vi "RRI LoadGo - Electromagnet.vi"(5 "Control Coils":T1(ring), 6 "Hardware Parameters":T2={"Scan Calibration [G/V]"=0.0, "Modulation Calibration [G/V]"=0.0, "Modulation Phase [deg]"=0.0, "Modulation Frequency [Hz]"=0.0, "Attenuation [dB]"=0, "Input Channel Count"=0, "Time constant"=7, "Sensitivity"=17, "Frequency Output Voltage [V]"=0.0, "Phase Output Voltage [V]"=0.0, "Lock-in Offset Compensation"=FALSE, "RF [GHz]"=0.0, "Q Start"=0.0, "Q End"=0.0, "Balance"=0.0, "Phase Error"=0.0, "AFC Error"=0.0, "AFC"=FALSE, "Magnet Rotation"=FALSE, "Balance Scaling Factor"=1.0, "Phase Error Scaling Factor"=1.0, "AFC Error Scaling Factor"=1.0, "Frequency Counter ID"="", "Sweep Waveform"=enum."Sawtooth", "Q-Factor Scale"=0.0, " Q-Data Scale"=0.0, " Q-Data Offset"=0.0, "Magnet Rotation Slope"=0.0, "Magnet Rotation Offset"=0.0, "Phase Sweep Resolution"=0.0, "Hardware Version Number"="", "Spectrometer ID Number"=0, "Spectrometer Name"="", "Lock in Saturation"=0.0, "Balance Threshold"=0.0, "Phase Error Threshold"=0.0, "AFC Error Threshold"=0.0, "Linear Actuator Length"=0.0, "Lock-in OK?"=FALSE, "Ignore Lock-in Comm. Failure"=FALSE, "Gradient Addresses"=[], "Gradient Calibrations [G/A*mm]"=[], "Gradient Power Supplies"=[], "Lock-in Address"="", "Magnet Type"=enum."RRI", "Camera Names"=[], "Sweep Limit [Gauss]"=0.0, "Modulation Limit [Gauss]"=0.0, "Balance Threshold Exceeded?"=FALSE, "Phase Threshold Exceeded?"=FALSE, "AFC Threshold Exceeded?"=FALSE, "Consecutive Re-tune attempts"=0, "Reverse Sweep Slope [sec]"=0.0, "Reverse Sweep Offset [G]"=0.0, "AFC Field Correction [V/MHz]"=0.0, "Active Gradients (X Y Z)"=[], "SpO2 Calibration [SpO2/V]"=1.0, "Heart Rate Calibration [BPM/V]"=1.0, "Thermocouple Channel"=""} {"Sensitivity" items=["", "2 nV", "5 nV", "10 nV", "20 nV", "50 nV", "100 nV", "200 nV", "500 nV", "1 uV", "2 uV", "5 uV", "10 uV", "20 uV", "50 uV", "100 uV", "200 uV", "500 uV", "1 mV", "2 mV", "5 mV", "10 mV", "20 mV", "50 mV", "100 mV", "200 mV", "500 mV", "1 V"]; "Time constant" items=["10 us", "20 us", "40 us", "80 us", "160 us", "320 us", "640 us", "5 ms", "10 ms", "20 ms", "50 ms", "100 ms", "200 ms", "500 ms", "1 s", "2 s", "5 s", "10 s", "20 s", "50 s", "100 s", "200 s", "500 s", "1 ks", "2 ks", "5 ks", "10 ks", "20 ks", "50 ks", "100 ks"]}, 7 "Acquisition Parameters":T3={"Magnet Angle [deg]"=0.0, "Magnet Angles [deg]"=[], "DeltaVpp [v]"=0.0, "SEM [v]"=0.0, "DeltaVpp Thresh [v]"=0.0, "SEM Thresh [v]"=0.0, "Adaptive Processing"=FALSE, "Acquire Q"=FALSE, "Acquire Photos"=FALSE, "Adaptive Tuning"=FALSE, "Automated Matching"=FALSE, "X-Gradient [G/mm]"=0.0, "Y-Gradient [G/mm]"=0.0, "Z-Gradient [G/mm]"=0.0, "Central Field [G]"=0.0, "Scan Width [G]"=0.0, "Mod. Amp. [G]"=0.0, "Scan Time [s]"=0.0, "Pre-Scan Delay [ms]"=0, "Measurement Timeout [s]"=0.0, "Electromagnet Main Field [G]"=0.0, "Locked Central Field [G]"=0.0, "Scans Excluded"=0, "Scans Completed"=0, "No. Scans/Set"=0, "No. Scans for SNR"=0, "Field Locked Frequency [GHz]"=0.0, "Auto Set-based Field Center"=FALSE, "Prompt for oxy acquisition updates"=FALSE, "Oxy QA Scan?"=FALSE, "Exclude Bad Data"=FALSE, "Optimizing RF Power"=FALSE, "Gradients on/off"=FALSE, "Running Script"=TRUE, "Opto-Coupler Current [A]"=0.0, "Continuous Sweeping"=FALSE, "Sweep Rise Time [sec]"=0, "Reverse Sweep Central Field [G]"=0.0, "Forward Sweep Central Field [G]"=0.0, "Sweep Calibrated"=FALSE, "Modulation Calibrated"=FALSE, "First CheckCal Scan?"=FALSE, "AFC Field Correction"=FALSE, "OxyQAInit Scan Width [G]"=0.0, "OxyQAInit Mod. Amp. [G]"=0.0, "Scans Completed/Session"=0, "Acquire SpO2"=FALSE, "Acquire Temperature"=FALSE, "Over Mod"=FALSE} {"OxyQAInit Mod. Amp. [G]" min=0.0; "OxyQAInit Scan Width [G]" min=0.0; "Mod. Amp. [G]" min=0.0; "Scan Width [G]" min=0.0; "Measurement Timeout [s]" min=0.0; "Scan Time [s]" min=0.0; "Z-Gradient [G/mm]" min=0.0; "Y-Gradient [G/mm]" min=0.0; "X-Gradient [G/mm]" min=0.0; "SEM Thresh [v]" min=0.0; "DeltaVpp Thresh [v]" min=0.0; "SEM [v]" min=0.0}) -> (0 "error out":errorcluster)   [LabVIEW 2016]
uses:
  Types/Acquisition Parameters.ctl
  Types/Hardware Parameters.ctl
  <vilib>/Instr/_visa.llb/VISA Configure Serial Port (Instr).vi
panel:
  # "Bridge I/O"
  # "Magnet Rotation"
  # "Field Calibration"
  # "Lock In Amplifier"
  # "Spectrometer Information"
  # "DAQ Settings"
  # "Gradient Coils and Field"
  # "X"
  # "Y"
  # "Z"
  # "Q-Measurements"
  # "Gradients"
  # "Field"
  # "Scans and Sets"
  # "Timing"
  # "Adaptive Dosimetric \nData Processing"
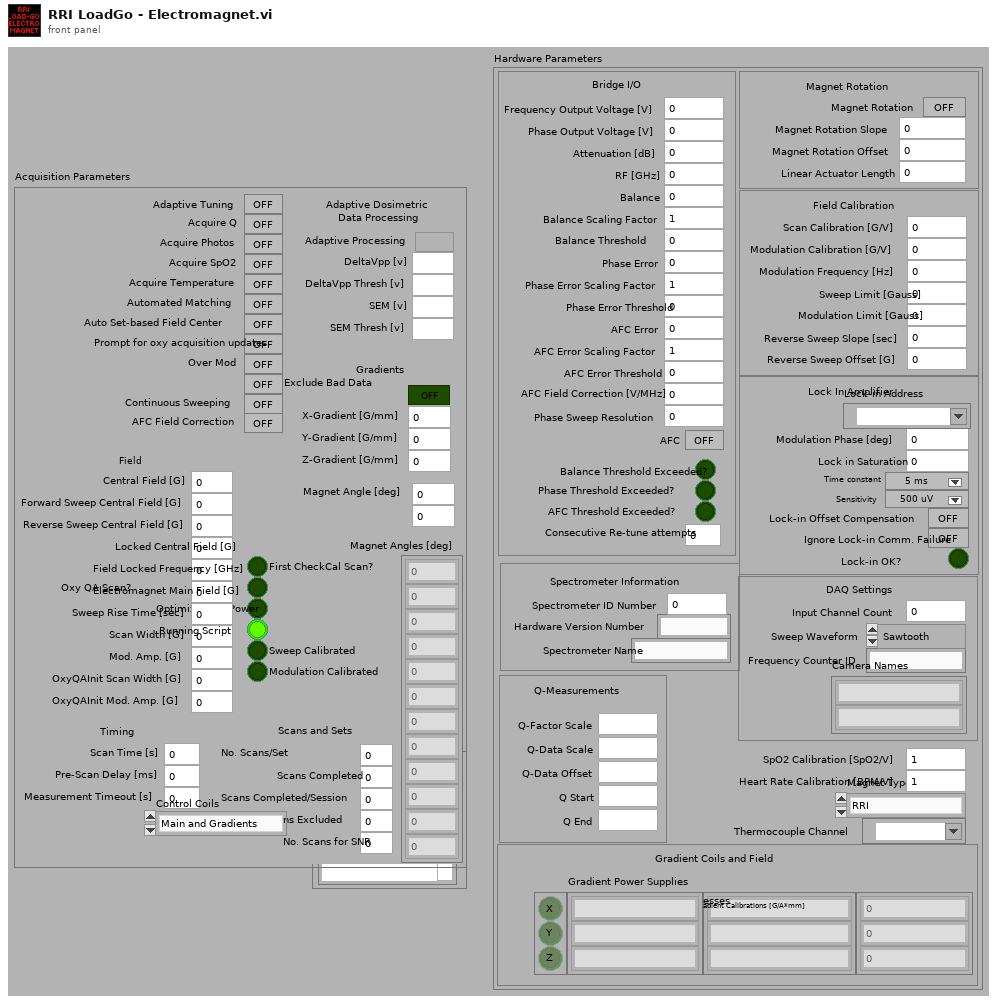
[diagram p1: front panel]
types:
  T1 = enum16{"Main and Gradients", "Main Field", "Gradients"}
  T2 = typedef "Hardware Parameters.ctl" = cluster{"Scan Calibration [G/V]":dbl, "Modulation Calibration [G/V]":dbl, "Modulation Phase [deg]":dbl, "Modulation Frequency [Hz]":dbl, "Attenuation [dB]":u16, "Input Channel Count":i32, "Time constant":u16, "Sensitivity":u16, "Frequency Output Voltage [V]":dbl, "Phase Output Voltage [V]":dbl, "Lock-in Offset Compensation":bool, "RF [GHz]":dbl, "Q Start":dbl, "Q End":dbl, "Balance":dbl, "Phase Error":dbl, "AFC Error":dbl, "AFC":bool, "Magnet Rotation":bool, "Balance Scaling Factor":dbl, "Phase Error Scaling Factor":dbl, "AFC Error Scaling Factor":dbl, "Frequency Counter ID":string, "Sweep Waveform":enum16{"Sine Wave", "Square Wave", "Sawtooth", "Triangle Wave"}, "Q-Factor Scale":dbl, " Q-Data Scale":dbl, " Q-Data Offset":dbl, "Magnet Rotation Slope":dbl, "Magnet Rotation Offset":dbl, "Phase Sweep Resolution":dbl, "Hardware Version Number":string, "Spectrometer ID Number":i32, "Spectrometer Name":string, "Lock in Saturation":dbl, "Balance Threshold":dbl, "Phase Error Threshold":dbl, "AFC Error Threshold":dbl, "Linear Actuator Length":dbl, "Lock-in OK?":bool, "Ignore Lock-in Comm. Failure":bool, "Gradient Addresses":string[], "Gradient Calibrations [G/A*mm]":dbl[], "Gradient Power Supplies":string[], "Lock-in Address":refnum<visa-resource-name>, "Magnet Type":enum16{"RRI", "BARDA", "Whole Body Permanent", "RRI Electromagnet"}, "Camera Names":string[], "Sweep Limit [Gauss]":dbl, "Modulation Limit [Gauss]":dbl, "Balance Threshold Exceeded?":bool, "Phase Threshold Exceeded?":bool, "AFC Threshold Exceeded?":bool, "Consecutive Re-tune attempts":i32, "Reverse Sweep Slope [sec]":dbl, "Reverse Sweep Offset [G]":dbl, "AFC Field Correction [V/MHz]":dbl, "Active Gradients (X Y Z)":bool[], "SpO2 Calibration [SpO2/V]":dbl, "Heart Rate Calibration [BPM/V]":dbl, "Thermocouple Channel":tag}
  T3 = typedef "Acquisition Parameters.ctl" = cluster{"Magnet Angle [deg]":dbl, "Magnet Angles [deg]":dbl[], "DeltaVpp [v]":dbl, "SEM [v]":dbl, "DeltaVpp Thresh [v]":dbl, "SEM Thresh [v]":dbl, "Adaptive Processing":bool, "Acquire Q":bool, "Acquire Photos":bool, "Adaptive Tuning":bool, "Automated Matching":bool, "X-Gradient [G/mm]":dbl, "Y-Gradient [G/mm]":dbl, "Z-Gradient [G/mm]":dbl, "Central Field [G]":dbl, "Scan Width [G]":dbl, "Mod. Amp. [G]":dbl, "Scan Time [s]":dbl, "Pre-Scan Delay [ms]":u32, "Measurement Timeout [s]":dbl, "Electromagnet Main Field [G]":dbl, "Locked Central Field [G]":dbl, "Scans Excluded":u32, "Scans Completed":u32, "No. Scans/Set":u32, "No. Scans for SNR":u32, "Field Locked Frequency [GHz]":dbl, "Auto Set-based Field Center":bool, "Prompt for oxy acquisition updates":bool, "Oxy QA Scan?":bool, "Exclude Bad Data":bool, "Optimizing RF Power":bool, "Gradients on/off":bool, "Running Script":bool, "Opto-Coupler Current [A]":dbl, "Continuous Sweeping":bool, "Sweep Rise Time [sec]":u32, "Reverse Sweep Central Field [G]":dbl, "Forward Sweep Central Field [G]":dbl, "Sweep Calibrated":bool, "Modulation Calibrated":bool, "First CheckCal Scan?":bool, "AFC Field Correction":bool, "OxyQAInit Scan Width [G]":dbl, "OxyQAInit Mod. Amp. [G]":dbl, "Scans Completed/Session":u32, "Acquire SpO2":bool, "Acquire Temperature":bool, "Over Mod":bool}
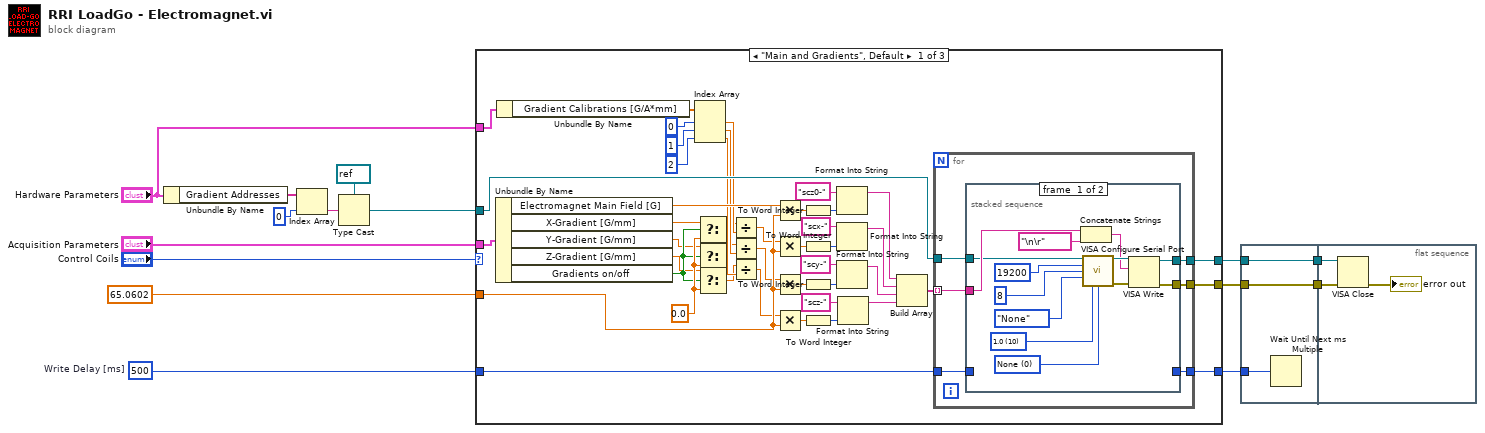
[diagram p0: block diagram]
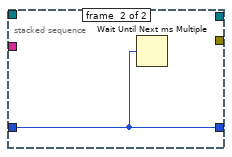
[diagram p2: hidden frame]
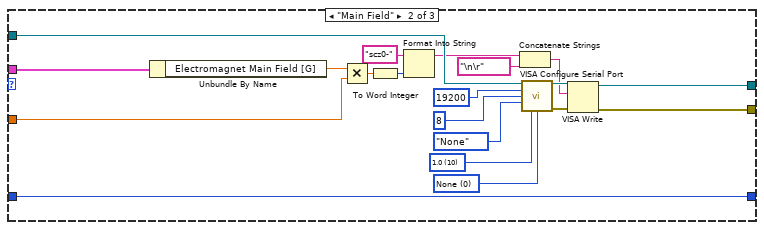
[diagram p3: hidden frame]
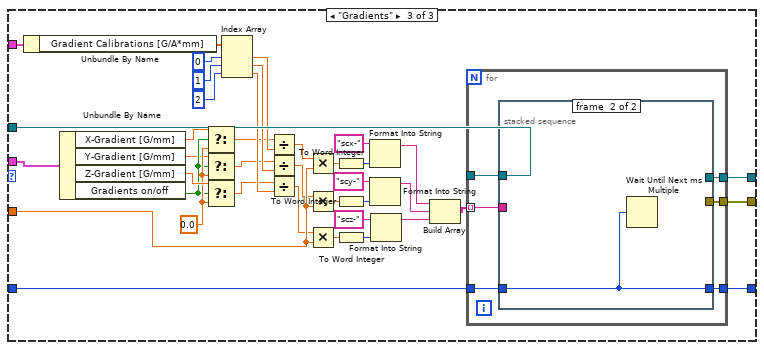
[diagram p4: hidden frame]
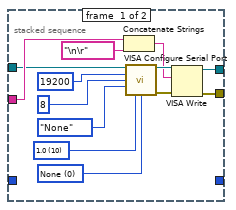
[diagram p5: hidden frame]
diagram:
  w2 = u32 500  # Write Delay [ms]
  n1 = Unbundle By Name("Hardware Parameters") -> ("Gradient Addresses"=w9:string[])
  n2 = Index Array(array=w9, index=0) -> (element=w11:string)
  n3 = Type Cast(type=refnum<visa-resource-name> refnum ("VISA resource name"), x=w11) -> (*(type *) &x=w7:refnum<visa-resource-name>)
  n4 = case shown="\"Main and Gradients\", Default" "Control Coils" {
    tunnel: "Acquisition Parameters" -> [w42 w95 w125]
    tunnel: [w40 w94 w122] -> w13
    tunnel: [w39 w93 w121] -> w12
    tunnel: w7 -> [w38 w92 w124]
    tunnel: 65.0602 ("y") -> [w37 w81 w123]
    tunnel: [w36 w80 w120] -> w3
    tunnel: w2 -> [w35 w80 w119]
    tunnel: "Hardware Parameters" -> [w30 _ w117]
    frame "Main and Gradients", Default {
      w23 = 0.0 ("f")
      n5 = Unbundle By Name(w42) -> ("Electromagnet Main Field [G]"=w41:dbl, "X-Gradient [G/mm]"=w21:dbl, "Y-Gradient [G/mm]"=w20:dbl, "Z-Gradient [G/mm]"=w19:dbl, "Gradients on/off"=w22:bool)
      n6 = Unbundle By Name(w30) -> ("Gradient Calibrations [G/A*mm]"=w34:dbl[])
      n7 = Index Array(array=w34, index #1=0 ("index"), index #2=1 ("index"), index #3=2 ("index")) -> (element #1=w26:dbl, element #2=w25:dbl, element #3=w24:dbl)
      n8 = Select(t=w21, s=w22, f=w23) -> (s? t:f=w18:dbl)
      n9 = Select(t=w20, s=w22, f=w23) -> (s? t:f=w17:dbl)
      n10 = Select(t=w19, s=w22, f=w23) -> (s? t:f=w16:dbl)
      n11 = Divide(x=w18, y=w26) -> (x/y=w29:dbl)
      n12 = Divide(x=w17, y=w25) -> (x/y=w28:dbl)
      n13 = Divide(x=w16, y=w24) -> (x/y=w27:dbl)
      n14 = Multiply(x=w41, y=w37) -> (x*y=w59:dbl)
      n15 = Multiply(x=w29, y=w37) -> (x*y=w56:dbl)
      n16 = Multiply(x=w28, y=w37) -> (x*y=w54:dbl)
      n17 = Multiply(x=w27, y=w37) -> (x*y=w52:dbl)
      n18 = To Word Integer(number=w59) -> (16bit integer=w58:i16)
      n19 = To Word Integer(number=w56) -> (16bit integer=w55:i16)
      n20 = To Word Integer(number=w54) -> (16bit integer=w53:i16)
      n21 = To Word Integer(number=w52) -> (16bit integer=w51:i16)
      n22 = Format Into String(initial string="scz0-" ("string main"), w58) -> (resulting string=w57:string)  [unwired: 2 in, 1 out]
      n23 = Format Into String(initial string="scx-" ("initial X-Grad"), w55) -> (resulting string=w50:string)  [unwired: 2 in, 1 out]
      n24 = Format Into String(initial string="scy-" ("initial Y-Grad"), w53) -> (resulting string=w49:string)  [unwired: 2 in, 1 out]
      n25 = Format Into String(initial string="scz-" ("initial Z-Grad"), w51) -> (resulting string=w48:string)  [unwired: 2 in, 1 out]
      n26 = Build Array(w57, w50, w49, w48) -> (w47:string[])
      n27 = for {
        tunnel: w47 -> [w65] mode=indexing
        tunnel: [w64] -> w39
        tunnel: [w63] -> w40
        tunnel: w38 -> [w62]
        tunnel: [w61] -> w36
        tunnel: w35 -> [w60]
        n28 = stacked-sequence {
          tunnel: w65 -> [w75 _]
          tunnel: [w72 _] -> w64
          tunnel: [w67 _] -> w63
          tunnel: w62 -> [w66 _]
          tunnel: [_ w79] -> w61
          tunnel: w60 -> [_ w79]
          frame #0 {
            w68 = u16 0 items=["None", "XON/XOFF", "RTS/CTS", "XON/XOFF & RTS/CTS", "DTR/DSR", "XON/XOFF & DTR/DSR"] ("flow control (0:none)")
            w69 = u16 10 items=["1.0"=10, "1.5"=15, "2.0"=20] ("stop bits (10: 1 bit)")
            n29 = Concatenate Strings(w75, "\n\r") -> (w74:string)
            n30 = call-poly "VISA Configure Serial Port"("VISA resource name"=w66, "baud rate (9600)"=u32 19200, "data bits (8)"=u16 8, "parity (0:none)"=enum16{"None", "Odd", "Even", "Mark", "Space"}."None", "stop bits (10: 1 bit)"=w69, "flow control (0:none)"=w68) -> ("VISA resource name out"=w77:refnum<visa-resource-name>, "error out"=w78:errorcluster)  [unwired: 1 in, 7 out]
            n31 = VISA Write(VISA resource name=w77, write buffer=w74, error in (no error)=w78) -> (VISA resource name out=w67:refnum<visa-resource-name>, error out=w72:errorcluster)  [unwired: 1 out]
          }
          frame #1 {
            n32 = Wait Until Next ms Multiple(millisecond multiple=w79) -> ()  [unwired: 1 out]
          }
        }
      }
    }
    frame "Main Field" {
      w82 = u16 0 items=["None", "XON/XOFF", "RTS/CTS", "XON/XOFF & RTS/CTS", "DTR/DSR", "XON/XOFF & DTR/DSR"] ("flow control (0:none)")
      w83 = u16 10 items=["1.0"=10, "1.5"=15, "2.0"=20] ("stop bits (10: 1 bit)")
      n33 = Unbundle By Name(w95) -> ("Electromagnet Main Field [G]"=w96:dbl)
      n34 = Multiply(x=w96, y=w81) -> (x*y=w99:dbl)
      n35 = To Word Integer(number=w99) -> (16bit integer=w98:i16)
      n36 = Format Into String(initial string="scz0-" ("string main"), w98) -> (resulting string=w91:string)  [unwired: 2 in, 1 out]
      n37 = Concatenate Strings(w91, "\n\r") -> (w87:string)
      n38 = call-poly "VISA Configure Serial Port"("VISA resource name"=w92, "baud rate (9600)"=u32 19200, "data bits (8)"=u16 8, "parity (0:none)"=enum16{"None", "Odd", "Even", "Mark", "Space"}."None", "stop bits (10: 1 bit)"=w83, "flow control (0:none)"=w82) -> ("VISA resource name out"=w89:refnum<visa-resource-name>, "error out"=w90:errorcluster)  [unwired: 1 in, 7 out]
      n39 = VISA Write(VISA resource name=w89, write buffer=w87, error in (no error)=w90) -> (VISA resource name out=w94:refnum<visa-resource-name>, error out=w93:errorcluster)  [unwired: 1 out]
    }
    frame "Gradients" {
      w106 = 0.0 ("f")
      n40 = Unbundle By Name(w117) -> ("Gradient Calibrations [G/A*mm]"=w118:dbl[])
      n41 = Unbundle By Name(w125) -> ("X-Gradient [G/mm]"=w100:dbl, "Y-Gradient [G/mm]"=w101:dbl, "Z-Gradient [G/mm]"=w107:dbl, "Gradients on/off"=w102:bool)
      n42 = Select(t=w100, s=w102, f=w106) -> (s? t:f=w105:dbl)
      n43 = Select(t=w101, s=w102, f=w106) -> (s? t:f=w104:dbl)
      n44 = Select(t=w107, s=w102, f=w106) -> (s? t:f=w103:dbl)
      n45 = Index Array(array=w118, index #1=0 ("index"), index #2=1 ("index"), index #3=2 ("index")) -> (element #1=w113:dbl, element #2=w112:dbl, element #3=w111:dbl)
      n46 = Divide(x=w105, y=w113) -> (x/y=w110:dbl)
      n47 = Divide(x=w104, y=w112) -> (x/y=w109:dbl)
      n48 = Divide(x=w103, y=w111) -> (x/y=w108:dbl)
      n49 = Multiply(x=w110, y=w123) -> (x*y=w138:dbl)
      n50 = Multiply(x=w109, y=w123) -> (x*y=w136:dbl)
      n51 = Multiply(x=w108, y=w123) -> (x*y=w134:dbl)
      n52 = To Word Integer(number=w138) -> (16bit integer=w137:i16)
      n53 = To Word Integer(number=w136) -> (16bit integer=w135:i16)
      n54 = To Word Integer(number=w134) -> (16bit integer=w133:i16)
      n55 = Format Into String(initial string="scx-" ("initial X-Grad"), w137) -> (resulting string=w132:string)  [unwired: 2 in, 1 out]
      n56 = Format Into String(initial string="scy-" ("initial Y-Grad"), w135) -> (resulting string=w131:string)  [unwired: 2 in, 1 out]
      n57 = Format Into String(initial string="scz-" ("initial Z-Grad"), w133) -> (resulting string=w130:string)  [unwired: 2 in, 1 out]
      n58 = Build Array(w132, w131, w130) -> (w129:string[])
      n59 = for {
        tunnel: w129 -> [w144] mode=indexing
        tunnel: [w143] -> w121
        tunnel: [w142] -> w122
        tunnel: w124 -> [w141]
        tunnel: [w140] -> w120
        tunnel: w119 -> [w139]
        n60 = stacked-sequence {
          tunnel: w144 -> [w154 _]
          tunnel: [w151 _] -> w143
          tunnel: [w146 _] -> w142
          tunnel: w141 -> [w145 _]
          tunnel: [_ w158] -> w140
          tunnel: w139 -> [_ w158]
          frame #0 {
            w147 = u16 0 items=["None", "XON/XOFF", "RTS/CTS", "XON/XOFF & RTS/CTS", "DTR/DSR", "XON/XOFF & DTR/DSR"] ("flow control (0:none)")
            w148 = u16 10 items=["1.0"=10, "1.5"=15, "2.0"=20] ("stop bits (10: 1 bit)")
            n61 = Concatenate Strings(w154, "\n\r") -> (w153:string)
            n62 = call-poly "VISA Configure Serial Port"("VISA resource name"=w145, "baud rate (9600)"=u32 19200, "data bits (8)"=u16 8, "parity (0:none)"=enum16{"None", "Odd", "Even", "Mark", "Space"}."None", "stop bits (10: 1 bit)"=w148, "flow control (0:none)"=w147) -> ("VISA resource name out"=w156:refnum<visa-resource-name>, "error out"=w157:errorcluster)  [unwired: 1 in, 7 out]
            n63 = VISA Write(VISA resource name=w156, write buffer=w153, error in (no error)=w157) -> (VISA resource name out=w146:refnum<visa-resource-name>, error out=w151:errorcluster)  [unwired: 1 out]
          }
          frame #1 {
            n64 = Wait Until Next ms Multiple(millisecond multiple=w158) -> ()  [unwired: 1 out]
          }
        }
      }
    }
  }
  n65 = flat-sequence {
    tunnel: w12 -> [w160]
    tunnel: w13 -> [w161]
    tunnel: [w161] -> w5
    tunnel: [w160] -> w4
    tunnel: w3 -> [w159]
    tunnel: w5 -> [w163]
    tunnel: w4 -> [w162]
    frame #0 {
      n66 = Wait Until Next ms Multiple(millisecond multiple=w159) -> ()  [unwired: 1 out]
    }
    frame #1 {
      n67 = VISA Close(VISA resource name=w163, error in (no error)=w162) -> (error out=→"error out":errorcluster)
    }
  }
